vi "Open.vi"(8 "error in (no error)":errorcluster, 11 "Config-Sqlite in":refnum<class "Config-Sqlite.lvclass">) -> (0 "error out":errorcluster, 3 "Config-Sqlite out":refnum<class "Config-Sqlite.lvclass">)   [LabVIEW 2020, in "CDM-Config.lvlib" / "Config-Sqlite.lvclass"]
uses:
  Config-Sqlite.lvclass
  Config-Sqlite.lvclass/Config-Sqlite.ctl
  <vilib>/drjdpowell/SQLite Library/SQL Connection/Open (string).vi
  <vilib>/AdvancedString/Path To Command Line String.vi
  <vilib>/drjdpowell/SQLite Library/SQL Connection/Connection.lvclass
  <vilib>/drjdpowell/SQLite Library/SQL Connection/Open (path).vi
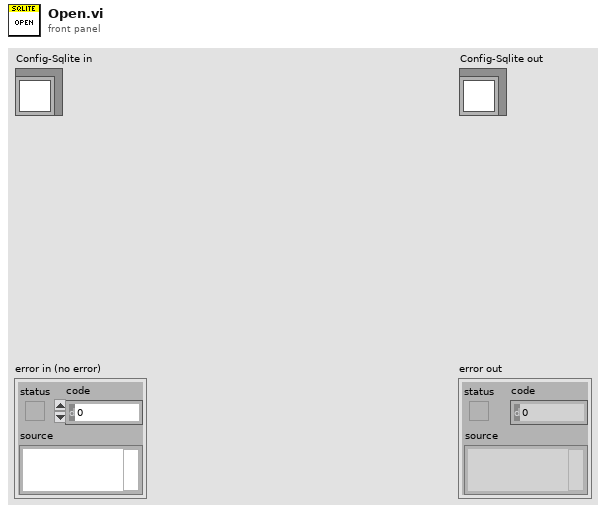
[diagram p1: front panel]
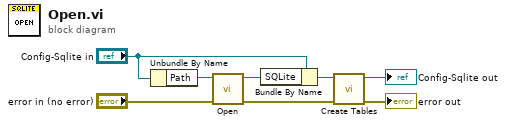
[diagram p0: block diagram]
diagram:
  n1 = Unbundle By Name("Config-Sqlite in") -> ("Path"=w5:path)
  n2 = call-poly <vilib>:"Open.vi"("error in (no error)"="error in (no error)", "db file"=w5) -> ("error out"=w4:errorcluster, "SQLite Connection"=w6:refnum<class "Connection.lvclass">)  [unwired: 8 in]
  n3 = Bundle By Name(cluster="Config-Sqlite in", "SQLite"=w6) -> (w3:refnum<class "Config-Sqlite.lvclass">)
  n4 = call "Create Tables.vi"("error in (no error)"=w4, "Config-Sqlite in"=w3) -> ("error out"=→"error out":errorcluster, "Config-Sqlite out"=→"Config-Sqlite out":refnum<class "Config-Sqlite.lvclass">)  [unwired: 8 in]
